vi "Buscar proyectos.vi"(10 "String out":string, 11 "Proyectos":string[](array[string])) -> (3 "Proyecto":string)   [LabVIEW 2017]
uses:
  <vilib>/GPower/String/GPString.lvlib
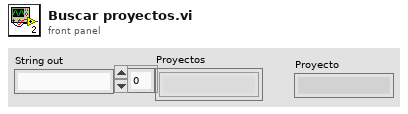
[diagram p1: front panel]
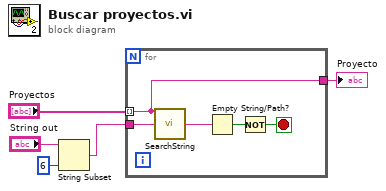
[diagram p0: block diagram]
diagram:
  n1 = String Subset(string="String out", length (rest)=6 ("length (rest)")) -> (substring=w2:string)  [unwired: 1 in]
  n2 = for {
    tunnel: "Proyectos" -> [w6] mode=indexing
    tunnel: w2 -> [w10]
    tunnel: [w6] -> w1
    stop <- w7 stop-if-true
    n3 = call <vilib>:"SearchString.vi"("String"=w6, "Search string"=w10) -> ("Rest of string"=w9:string)  [unwired: 11 in, 2 out]
    n4 = Empty String/Path?(string/path=w9) -> (empty?=w8:bool)
    n5 = Not(x=w8) -> (.not. x?=w7:bool)
  }
  "Proyecto" <- w1
